vi "Main On Compile Action VI.vi"(8 "error in (no error)":errorcluster, 11 "Device Item Ref in":T1 format="%.0x") -> (0 "error out":errorcluster)   [LabVIEW 2019, in "Ballard Arinc-429 System Explorer.lvlib"]
uses:
  Ballard Arinc-429 System Explorer.lvlib
  <vilib>/NI VeriStand/Custom Device API/Custom Device Item Ref.ctl
  Shared/Controls and Global/Compiled.Settings.ctl
  Shared/Controls and Global/RT HW Channel.ctl
  Shared/Controls and Global/RT Label Settings.ctl
  Shared/Controls and Global/Label.ctl
  Shared/Controls and Global/transferPeriod.ctl
  Shared/Controls and Global/RT Word Settings.ctl
  Shared/Controls and Global/RT Param Setting.ctl
  Shared/Controls and Global/Start Bit.ctl
  Shared/Controls and Global/Number of Bits.ctl
  <vilib>/NI VeriStand/Custom Device API/Block Data Reference.ctl
  <vilib>/NI VeriStand/Custom Device API/Data Reference.ctl
  Shared/Controls and Global/TransferType.ctl
  Shared/Controls and Global/Global.vi
  <vilib>/NI VeriStand/Custom Device API/Set Item Property (Variant).vi
  Shared/Ballard Arinc-429 Shared.lvlib
  <vilib>/NI VeriStand/Custom Device API/Custom Device API.lvlib
  <vilib>/NI/NIVS Inline Async API/_Data Access System Explorer/Data Access System Explorer.lvlib
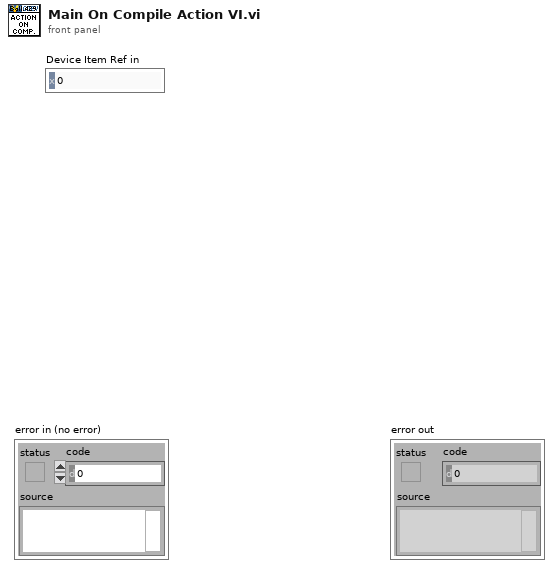
[diagram p1: front panel]
types:
  T1 = typedef "Custom Device API.lvlib/Custom Device Item Ref.ctl" = u64
  T2 = typedef "Ballard Arinc-429 Shared.lvlib/Compiled.Settings.ctl" = cluster{"Name":string, "Rx Config":T3[], "Tx Config":T3[]}
  T3 = typedef "Ballard Arinc-429 Shared.lvlib/RT HW Channel.ctl" = cluster{"Labels Settings":T4[], "channel handle":u64, "channel #":u16}
  T4 = typedef "Ballard Arinc-429 Shared.lvlib/RT Label Settings.ctl" = cluster{"Name":string, "xmlName":string, "Label":T5, "transferPeriod":T6, "SDI_Enabled":bool, "SDI":u8, "Word":T7, "TransferType":T13, "has timestamp?":bool, "Label Disable/Trigger Channel Reference":T1, "Message Handle":u64, "Initialized?":bool, "Word Initial Raw Value":u32, "Label Timestamp Channel Data Reference":T12}
  T5 = typedef "Ballard Arinc-429 Shared.lvlib/Label.ctl" = u8
  T6 = typedef "Ballard Arinc-429 Shared.lvlib/transferPeriod.ctl" = u32
  T7 = typedef "Ballard Arinc-429 Shared.lvlib/RT Word Settings.ctl" = cluster{"Param Setting":T8}
  T8 = typedef "Ballard Arinc-429 Shared.lvlib/RT Param Setting.ctl" = cluster{"Start Bit":T9[], "Num Bits":T10[], "Signed?":bool[], "ScaleFac":dbl[], "ScaleOffset":dbl[], "Block Data Refs":T11[], "Encoding":enum16{"BNR", "BCD", "Discrete"}[], "Values Array":dbl[], "Item Refs":T1[]}
  T9 = typedef "Ballard Arinc-429 Shared.lvlib/Start Bit.ctl" = i32
  T10 = typedef "Ballard Arinc-429 Shared.lvlib/Number of Bits.ctl" = i32
  T11 = typedef "Custom Device API.lvlib/Block Data Reference.ctl" = cluster{"Data Reference":T12, "Offset":u64, "Length":u64}
  T12 = typedef "Custom Device API.lvlib/Data Reference.ctl" = i32
  T13 = typedef "Ballard Arinc-429 Shared.lvlib/TransferType.ctl" = enum16{"ScheduledLabel", "Acyclic", "Block", "Strobe"}
  T14 = typedef "Custom Device API.lvlib/Custom Device Item Info.ctl" = cluster{"Name":string, "Is Channel":bool, "GUID":string, "Is Waveform":bool}
  T15 = cluster{"Name":string, "Type":enum16{"Output/Write", "Input/Read", "Input/ReadWrite"}, "VS Refs":T1[]}
  T16 = cluster{"Name":string, "Type":enum16{"Output/Write", "Input/Read", "Input/ReadWrite"}, "VS Refs":T1[]}[]
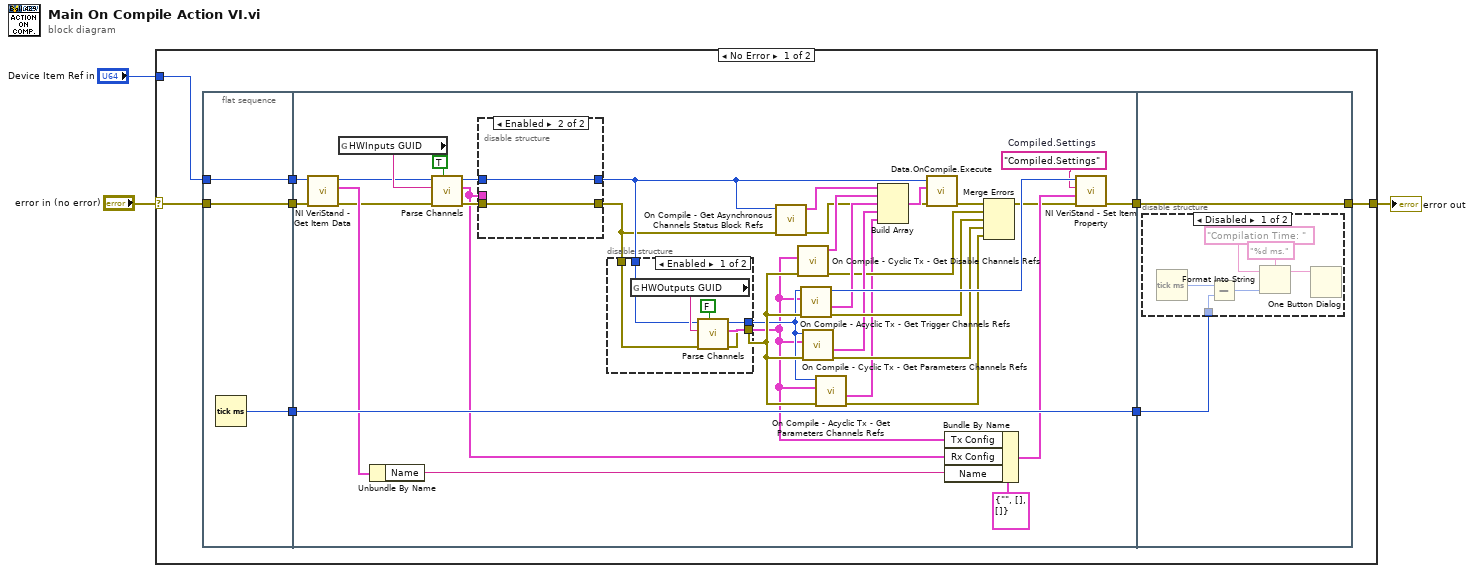
[diagram p0: block diagram]
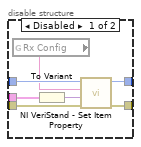
[diagram p2: hidden frame]
diagram:
  n1 = case shown="No Error" "error in (no error)" {
    selector: "error in (no error)" -> [w11 w76]
    tunnel: [w9 w76] -> w3
    tunnel: "Device Item Ref in" -> [w10 _]
    frame No Error {
      n2 = flat-sequence {
        tunnel: w11 -> [w13]
        tunnel: w10 -> [w14]
        tunnel: [w14] -> w8
        tunnel: [w13] -> w7
        tunnel: [w12] -> w6
        tunnel: w8 -> [w42]
        tunnel: w7 -> [w43]
        tunnel: w6 -> [w46]
        tunnel: [w46] -> w5
        tunnel: [w38] -> w4
        tunnel: [w69] -> w9
        tunnel: w5 -> [w68]
        tunnel: w4 -> [w69]
        frame #0 {
          n3 = Tick Count (ms)() -> (millisecond timer value=w12:u32)
        }
        frame #1 {
          w36 = "Compiled.Settings"  # Compiled.Settings
          n4 = call <vilib>:"NI VeriStand - Get Item Data.vi"("error in (no error)"=w43, "Item Ref in"=w42) -> ("error out"=w27:errorcluster, "Item Info"=w44:T14, "Item Ref out"=w28:T1)  [unwired: 6 in, 1 out]
          n5 = global read "Global.vi" "HWInputs GUID"() -> (w49:string)
          n6 = Unbundle By Name(w44) -> ("Name"=w40:string)
          n7 = call "Parse Channels.vi"("Rx? (T:True, F: False (Tx))"=TRUE, "error in (no error)"=w27, "Section GUID"=w49, "Device Reference in"=w28) -> ("error out"=w47:errorcluster, "Channel Data []"=w35:T3[], "Device Reference out"=w48:T1)  [unwired: 5 in]
          n8 = disable-structure shown="Enabled" {
            disable-tunnel: w48 -> [w56 w57]
            disable-tunnel: w47 -> [w53 w58]
            disable-tunnel: w35 -> [w52 _]
            disable-tunnel: [w51 w57] -> w33
            disable-tunnel: [w50 w58] -> w31
            frame Disabled {
              n9 = global read "Global.vi" "Rx Config"() -> (w55:string)
              n10 = To Variant(anything=w52) -> (Variant=w54:variant)
              n11 = call-poly <vilib>:"NI VeriStand - Set Item Property.vi"("error in (no error)"=w53, "Value"=w54, "Property Name"=w55, "Item Ref in"=w56) -> ("error out"=w50:errorcluster, "Item Ref out"=w51:T1)  [unwired: 5 in, 1 out]
            }
            frame Enabled {
            }
          }
          n12 = disable-structure shown="Enabled" {
            disable-tunnel: [w64 w66] -> w18
            disable-tunnel: [w63 _] -> w17
            disable-tunnel: w33 -> [w59 w66]
            disable-tunnel: w31 -> [w60 w67]
            disable-tunnel: [w61 w67] -> w19
            frame Enabled {
              n13 = global read "Global.vi" "HWOutputs GUID"() -> (w65:string)
              n14 = call "Parse Channels.vi"("Rx? (T:True, F: False (Tx))"=FALSE, "error in (no error)"=w60, "Section GUID"=w65, "Device Reference in"=w59) -> ("error out"=w61:errorcluster, "Channel Data []"=w63:T3[], "Device Reference out"=w64:T1)  [unwired: 5 in]
            }
            frame Disabled {
            }
          }
          n15 = call "On Compile - Get Asynchronous Channels Status Block Refs.vi"("error in (no error)"=w31, "Item Ref"=w33) -> ("error out"=w20:errorcluster, "Async Status Channels Refs"=w34:T15)  [unwired: 8 in]
          n16 = call "On Compile - Cyclic Tx - Get Disable Channels Refs.vi"("error in (no error)"=w19, "Channel Data [] In"=w17) -> ("error out"=w21:errorcluster, "Async Status Channels Refs"=w26:T15)  [unwired: 8 in]
          n17 = call "On Compile - Acyclic Tx - Get Trigger Channels Refs.vi"("error in (no error)"=w19, "Channel Data [] In"=w17, "Item Ref In"=w18) -> ("error out"=w24:errorcluster, "Group"=w25:T15, "Item Ref Out"=w39:T1)  [unwired: 5 in, 1 out]
          n18 = call "On Compile - Cyclic Tx - Get Parameters Channels Refs.vi"("error in (no error)"=w19, "Channel Data [] In"=w17, "Item Ref In"=w18) -> ("error out"=w22:errorcluster, "Group"=w23:T15)  [unwired: 5 in, 2 out]
          n19 = call "On Compile - Acyclic Tx - Get Parameters Channels Refs.vi"("error in (no error)"=w19, "Channel Data [] In"=w17, "Item Ref In"=w18) -> ("error out"=w15:errorcluster, "Group"=w16:T15)  [unwired: 5 in, 2 out]
          n20 = Build Array(w34, w26, w25, w23, w16) -> (w29:T16)
          n21 = call <vilib>:"Data.OnCompile.Execute.vi"("error in"=w20, "VS Ref Groups"=w29, "Custom Device Ref"=w33) -> ("error out"=w30:errorcluster)  [unwired: 7 in, 1 out]
          n22 = Bundle By Name(cluster=T2 {"Name"="", "Rx Config"=[], "Tx Config"=[]} ("Compiled.Settings"), "Tx Config"=w17, "Rx Config"=w35, "Name"=w40) -> (w41:T2)
          n23 = Merge Errors(w30, w21, w24, w22, w15) -> (w32:errorcluster)
          n24 = call-poly <vilib>:"NI VeriStand - Set Item Property.vi"("error in (no error)"=w32, "Value"=w41, "Property Name"=w36, "Item Ref in"=w39) -> ("error out"=w38:errorcluster)  [unwired: 5 in, 2 out]
        }
        frame #2 {
          n25 = disable-structure shown="Disabled" {
            disable-tunnel: w68 -> [w74 _]
            frame Disabled {
              n26 = Tick Count (ms)() -> (millisecond timer value=w75:u32)
              n27 = Subtract(x=w75, y=w74) -> (x-y=w73:u32)
              n28 = Format Into String(format string="%d ms.", initial string="Compilation Time: ", w73) -> (resulting string=w72:string)  [unwired: 1 in, 1 out]
              n29 = One Button Dialog(message=w72) -> ()  [unwired: 1 in, 1 out]
            }
            frame Enabled {
            }
          }
        }
      }
    }
    frame Error {
    }
  }
  "error out" <- w3
